vi "calc_phase_map.vi"(4 "u8_ar_image_pixel_array":i16[][][](array[numeric]), 5 "image name":string="fringe") -> (0 "raw phase map array":u8[][](array[numeric]), 1 "phase map":T1(plugin-control))   [LabVIEW 2011]
uses:
  global_vars.vi
panel:
  in  "add":dbl
  in  "multi":dbl
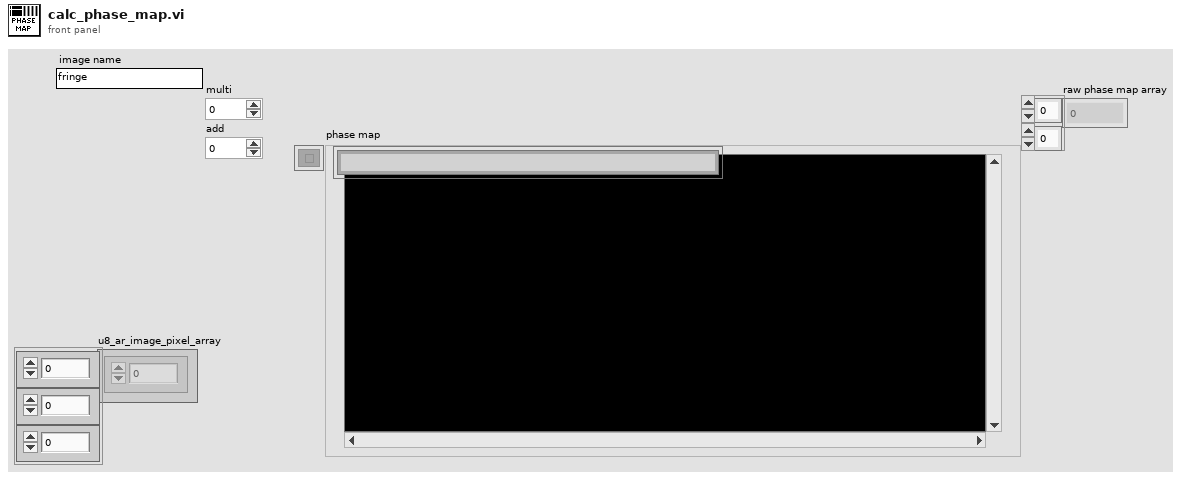
[diagram p1: front panel]
types:
  T1 = typedef "IMAQ Image.ctl" = refnum<image>
  T2 = typedef "Image Type" = u32
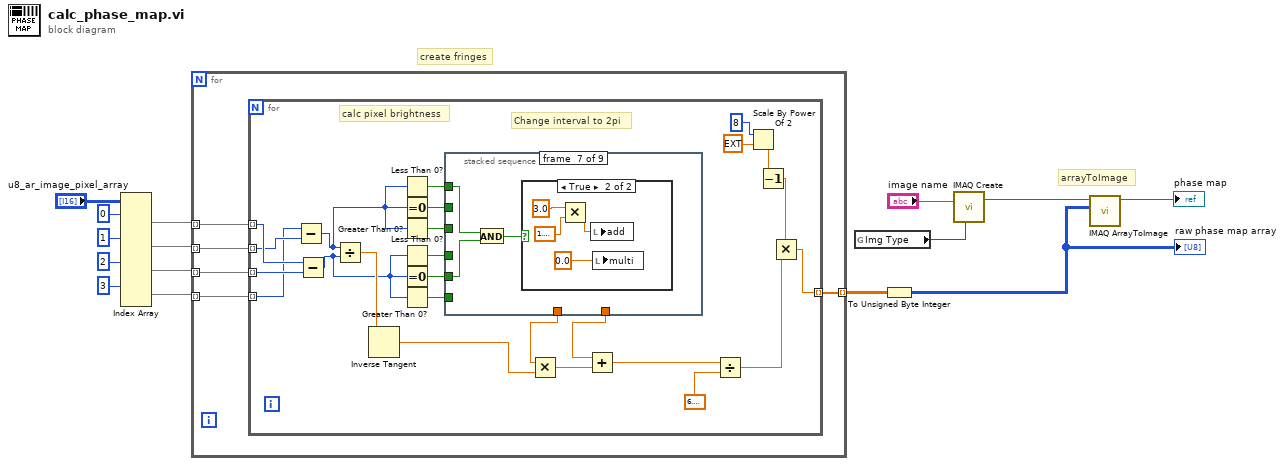
[diagram p0: block diagram]
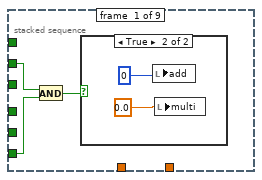
[diagram p2: hidden frame]
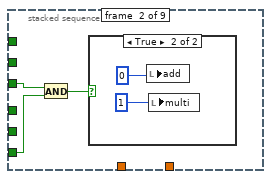
[diagram p4: hidden frame]
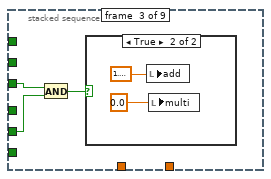
[diagram p6: hidden frame]
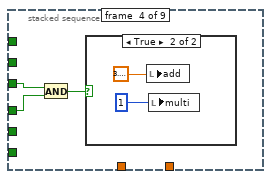
[diagram p8: hidden frame]
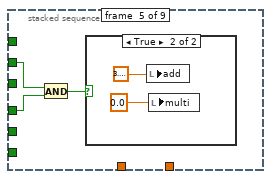
[diagram p10: hidden frame]
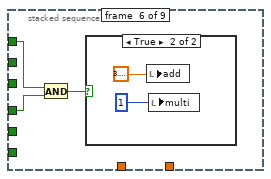
[diagram p12: hidden frame]
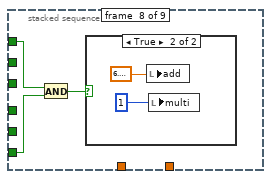
[diagram p15: hidden frame]
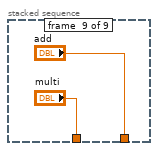
[diagram p17: hidden frame]
diagram:
  # "create fringes"
  # "arrayToImage"
  n1 = Index Array(array="u8_ar_image_pixel_array", index (dim 0) #1=0 ("index (page)"), index (dim 0) #2=1 ("index (page)"), index (dim 0) #3=2 ("index (page)"), index (dim 0) #4=3 ("index (page)")) -> (element #1=w9:i16[][], element #2=w8:i16[][], element #3=w7:i16[][], element #4=w6:i16[][])  [unwired: 8 in]
  n2 = for {
    tunnel: w9 -> [w20] mode=indexing
    tunnel: w8 -> [w19] mode=indexing
    tunnel: w7 -> [w18] mode=indexing
    tunnel: w6 -> [w17] mode=indexing
    tunnel: [w16] -> w5 mode=indexing
    n3 = for {
      tunnel: w20 -> [w31] mode=indexing
      tunnel: w19 -> [w30] mode=indexing
      tunnel: w18 -> [w29] mode=indexing
      tunnel: w17 -> [w28] mode=indexing
      tunnel: [w41] -> w16 mode=indexing
      # "Change interval to 2pi"
      # "calc pixel brightness"
      n4 = Subtract(x=w28, y=w30) -> (x-y=w26:i16)
      n5 = Subtract(x=w31, y=w29) -> (x-y=w25:i16)
      n6 = Divide(x=w26, y=w25) -> (x/y=w27:dbl)
      n7 = Inverse Tangent(1:w27) -> (0:w23:dbl)
      n8 = Less Than 0?(x=w26) -> (x < 0?=w38:bool)
      n9 = Equal To 0?(x=w26) -> (x = 0?=w37:bool)
      n10 = Greater Than 0?(x=w26) -> (x > 0?=w36:bool)
      n11 = Less Than 0?(x=w25) -> (x < 0?=w33:bool)
      n12 = Equal To 0?(x=w25) -> (x = 0?=w34:bool)
      n13 = Greater Than 0?(x=w25) -> (x > 0?=w35:bool)
      n14 = stacked-sequence {
        tunnel: w38 -> [_ _ _ _ _ w72 w77 w83 _]
        tunnel: w37 -> [w47 _ _ _ w67 _ _ _ _]
        tunnel: w36 -> [_ w52 w56 w62 _ _ _ _ _]
        tunnel: w35 -> [w46 w51 _ _ _ _ _ w84 _]
        tunnel: w34 -> [_ _ w57 _ _ _ w76 _ _]
        tunnel: w33 -> [_ _ _ w61 w66 w71 _ _ _]
        tunnel: [_ _ _ _ _ _ _ _ "add"] -> w24
        tunnel: [_ _ _ _ _ _ _ _ "multi"] -> w21
        frame #0 {
          n15 = And(x=w47, y=w46) -> (x .and. y?=w48:bool)
          n16 = case shown="True" w48 {
            frame False {
            }
            frame True {
              n17 = local write "add"(0) -> ()
              n18 = local write "multi"(0.0) -> ()
            }
          }
        }
        frame #1 {
          n19 = And(x=w52, y=w51) -> (x .and. y?=w53:bool)
          n20 = case shown="True" w53 {
            frame False {
            }
            frame True {
              n21 = local write "add"(0) -> ()
              n22 = local write "multi"(1) -> ()
            }
          }
        }
        frame #2 {
          n23 = And(x=w56, y=w57) -> (x .and. y?=w58:bool)
          n24 = case shown="True" w58 {
            frame False {
            }
            frame True {
              n25 = local write "add"(1.5707963267948966) -> ()
              n26 = local write "multi"(0.0) -> ()
            }
          }
        }
        frame #3 {
          n27 = And(x=w62, y=w61) -> (x .and. y?=w63:bool)
          n28 = case shown="True" w63 {
            frame False {
            }
            frame True {
              n29 = local write "add"(3.141592653589793) -> ()
              n30 = local write "multi"(1) -> ()
            }
          }
        }
        frame #4 {
          n31 = And(x=w67, y=w66) -> (x .and. y?=w68:bool)
          n32 = case shown="True" w68 {
            frame False {
            }
            frame True {
              n33 = local write "add"(3.141592653589793) -> ()
              n34 = local write "multi"(0.0) -> ()
            }
          }
        }
        frame #5 {
          n35 = And(x=w72, y=w71) -> (x .and. y?=w73:bool)
          n36 = case shown="True" w73 {
            frame False {
            }
            frame True {
              n37 = local write "add"(3.141592653589793) -> ()
              n38 = local write "multi"(1) -> ()
            }
          }
        }
        frame #6 {
          n39 = And(x=w77, y=w76) -> (x .and. y?=w78:bool)
          n40 = case shown="True" w78 {
            frame False {
            }
            frame True {
              n41 = Multiply(x=3.0, y=1.5707963267948966) -> (x*y=w81:dbl)
              n42 = local write "add"(w81) -> ()
              n43 = local write "multi"(0.0) -> ()
            }
          }
        }
        frame #7 {
          n44 = And(x=w83, y=w84) -> (x .and. y?=w85:bool)
          n45 = case shown="True" w85 {
            frame False {
            }
            frame True {
              n46 = local write "add"(6.283185307179586) -> ()
              n47 = local write "multi"(1) -> ()
            }
          }
        }
        frame #8 {
        }
      }
      n48 = Multiply(x=w21, y=w23) -> (x*y=w22:dbl)
      n49 = Add(x=w24, y=w22) -> (x+y=w32:dbl)
      n50 = Divide(x=w32, y=6.283185307179586) -> (x/y=w42:dbl)
      n51 = Scale By Power Of 2(n=8, x=ext 1.0) -> (x*2^n=w44:ext)
      n52 = Decrement(x=w44) -> (x-1=w43:ext)
      n53 = Multiply(x=w43, y=w42) -> (x*y=w41:ext)
    }
  }
  n54 = global read "global_vars.vi" "Img Type"() -> (w1:T2)
  n55 = To Unsigned Byte Integer(number=w5) -> (unsigned 8bit integer=w3:u8[][])
  "raw phase map array" <- w3
  n56 = call "IMAQ Create"("Image Name"="image name", "Image Type"=w1) -> ("New Image"=w2:T1)  [unwired: 2 in, 2 out]
  n57 = call "IMAQ ArrayToImage"("Image Pixels (U8)"=w3, "Image"=w2) -> ("Image Out"=→"phase map":T1)  [unwired: 8 in, 1 out]
